vi "UsrProfiles-Set user button.vi"(8 "error in (no error)":errorcluster) -> (0 "error out":errorcluster)   [LabVIEW 2020]
uses:
  Global Variables/gl_UI Ctrl Refs.vi
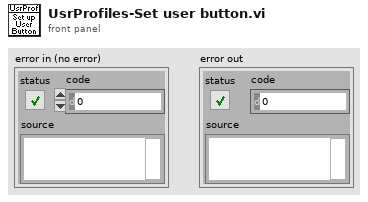
[diagram p1: front panel]
types:
  T1 = typedef "UI ctrl refs cluster.ctl" = cluster{"Top level VI path":path, "Top level VI ref":refnum<vi>, "User menu ref":refnum<k9>, "Sub Panel control":refnum<vi>, "Imaging Param Tab":refnum<vi>, "Occurrence-Start drivers":refnum<k4>, "Occurrence-Speed logging initialised":refnum<k4>, "Occurrence-XYZ stage initialised":refnum<k4>, "Exit button":refnum<vi>, "Status ind":refnum<vi>, "Set as origin":refnum<vi>, "Speed Logging":refnum<vi>, "Time Lapse":refnum<vi>, "Live Imaging":refnum<vi>, "AOL Z Stack":refnum<vi>, "Motor Z Stack":refnum<vi>, "Funct Acq button":refnum<vi>, "Hard Shutter":refnum<vi>, "Virtual Shutter":refnum<vi>, "Laser Power":refnum<vi>, "AOL Mode":refnum<vi>, "Frame Size":refnum<vi>, "Field of View":refnum<vi>, "Dwell Time":refnum<vi>, "Zoom":refnum<vi>, "AOL Z":refnum<vi>, "Objective":refnum<vi>, "Axis":refnum<vi>, "Paths & Names":refnum<vi>, "Experiment folder path (ind.)":refnum<vi>, "Last State (Ind.)":refnum<vi>, "Averages":refnum<vi>, "Angle (degrees)":refnum<vi>, "X centre":refnum<vi>, "Y centre":refnum<vi>, "Plane Mode":refnum<vi>, "# Planes":refnum<vi>, "Z Start":refnum<vi>, "Z Stop":refnum<vi>, "Z Step":refnum<vi>, "PMT 1":refnum<vi>, "PMT 2":refnum<vi>, "Stage XYZ Position":refnum<vi>, "Pockels@Z Start":refnum<vi>, "Pockels@Z Stop":refnum<vi>, "Obtain Z Start":refnum<vi>, "Obtain Z Stop":refnum<vi>, "Live stim.trig.period":refnum<vi>, "Live stim.trig.enable":refnum<vi>, "Movement Correction":refnum<vi>, "Load Reference Image":refnum<vi>, "XY Stage Move":refnum<vi>, "MovCor Cluster":refnum<vi>, "RefDAQParam":refnum<vi>, "Funct. Acq. Pockels Modulation":refnum<vi>, "Ref Laser Power":refnum<vi>, "Enable Video Recording":refnum<vi>, "Video Record-Live Imaging":refnum<vi>, "Video Record-Funct acq":refnum<vi>, "Reference Source":refnum<vi>, "AOL Z-stack Chirps Ready (ind)":refnum<vi>, "Target time between mov.cor. ref triggers (ms)":refnum<vi>, "Funct. Acq. Ref frame save":refnum<vi>, "Tracking button":refnum<vi>, "Show ref plots window":refnum<vi>, "Center freq ind (nm)":refnum<vi>, "Pickup mode (ind)":refnum<vi>, "Logging queue (ind)":refnum<vi>, "Back aperture power (ind.)":refnum<vi>, "Power after objective (ind.)":refnum<vi>, "Switch user":refnum<vi>, "Ls1 Conn. Status":refnum<vi>, "Ls1Tuning Status":refnum<vi>, "Ls1 Faults":refnum<vi>, "Ls1 Connection":refnum<vi>, "Ls1 Mode":refnum<vi>, "Ls1 POWER [mW]":refnum<vi>, "Ls1Shutter":refnum<vi>, "Ls1 Wavelength":refnum<vi>, "Ls1 Note":refnum<vi>, "Ls1 Confirm Wav":refnum<vi>, "Ls1 PreChrp Prism1":refnum<vi>, "Ls1 PreChrp Prism2":refnum<vi>, "Ls1 wav top Ind":refnum<vi>, "Ls1 power top Ind":refnum<vi>, "Ls1 Pump peak Hold":refnum<vi>, "Ls1 Status Ind":refnum<vi>, "Ls1 wav cancel":refnum<vi>, "Experiment Type":refnum<vi>, "Biology Information":refnum<vi>, "Camera recording status":refnum<vi>}
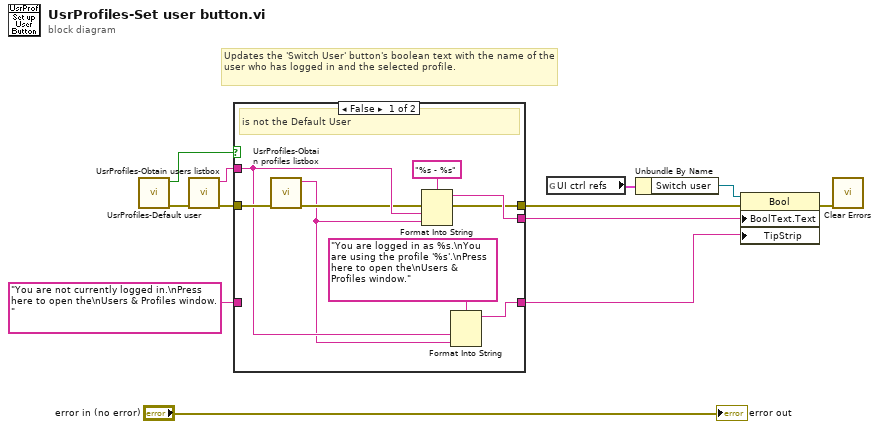
[diagram p0: block diagram]
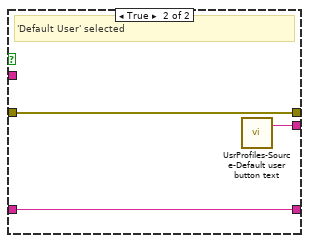
[diagram p2: hidden frame]
diagram:
  # "Updates the 'Switch User' button's boolean text with the name of the user who has logged in and the selected profile."
  n1 = call "UsrProfiles-Default user.vi"() -> ("error out"=w1:errorcluster, "Default user selected"=w2:bool)  [unwired: 9 in, 1 out]
  n2 = call "UsrProfiles-Obtain users listbox.vi"("error in (no error)"=w1) -> ("error out"=w4:errorcluster, "Selected user's name"=w3:string)  [unwired: 7 in, 2 out]
  n3 = case shown="False" w2 {
    tunnel: [w16 w22] -> w7
    tunnel: w4 -> [w21 w23]
    tunnel: [w14 w23] -> w12
    tunnel: w3 -> [w17 _]
    tunnel: [w19 w24] -> w5
    tunnel: "You are not currently logged in.\nPress here to open the\nUsers & Profiles window." ("Tip Strip") -> [_ w24]
    frame False {
      # "is not the Default User"
      n4 = call "UsrProfiles-Obtain profiles listbox.vi"("error in (no error)"=w21) -> ("error out"=w15:errorcluster, "Selected profile's name"=w13:string)  [unwired: 7 in, 2 out]
      n5 = Format Into String(format string="%s - %s", error in=w15, w17, w13) -> (resulting string=w16:string, error out=w14:errorcluster)  [unwired: 1 in]
      n6 = Format Into String(format string="You are logged in as %s.\nYou are using the profile '%s'.\nPress here to open the\nUsers & Profiles window." ("Tip Strip"), w17, w13) -> (resulting string=w19:string)  [unwired: 2 in, 1 out]
    }
    frame True {
      # "'Default User' selected"
      n7 = call "UsrProfiles-Source-Default user button text.vi"() -> ("Default user boolean text constant"=w22:string)  [unwired: 3 in]
    }
  }
  n8 = global read "gl_UI Ctrl Refs.vi" "UI ctrl refs"() -> (w11:T1)
  n9 = Unbundle By Name(w11) -> ("Switch user"=w10:refnum<vi>)
  n10 = property class="Bool"(reference=w10, error in=w12, "BoolText.Text"=w7, "TipStrip"=w5) -> (error out=w8:errorcluster)  [unwired: 1 out]
  n11 = call <vilib>:"Clear Errors.vi"("error in (no error)"=w8) -> ()  [unwired: 5 in, 2 out]
  "error out" <- "error in (no error)"
